vi "Sequence.BuildChannelLookup.vi"(8 "error in (no error)":errorcluster, 10 "Output Channels":T1[](array[typedef]), 11 "ChannelLookup":variant) -> (0 "error out":errorcluster, 3 "ChannelLookup":variant)   [LabVIEW 2013, in "Simple Sequence Editor.lvlib"]
uses:
  Simple Sequence Editor.lvlib
  Types/ChannelProperties.ctl
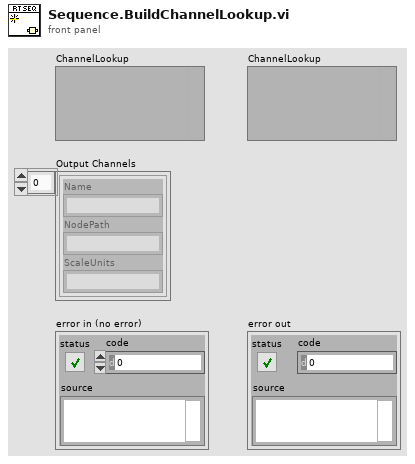
[diagram p1: front panel]
types:
  T1 = typedef "Simple Sequence Editor.lvlib/ChannelProperties.ctl" = cluster{"Name":string, "NodePath":string, "ScaleUnits":string}
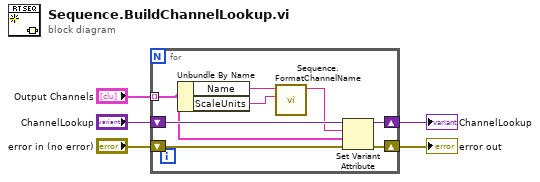
[diagram p0: block diagram]
diagram:
  n1 = for {
    shift-right: [w12] -> w5
    shift-left: "ChannelLookup" -> [w13]
    shift-right: [w11] -> w4
    shift-left: "error in (no error)" -> [w10]
    tunnel: "Output Channels" -> [w9] mode=indexing
    n2 = Unbundle By Name(w9) -> ("Name"=w7:string, "ScaleUnits"=w8:string)
    n3 = call "Sequence.FormatChannelName.vi"("ScaleUnits"=w8, "Name"=w7) -> ("String"=w6:string)  [unwired: 9 in]
    n4 = Set Variant Attribute(Variant=w13, name=w6, value=w9, error in=w10) -> (Variant out=w12:variant, error out=w11:errorcluster)  [unwired: 1 out]
  }
  "ChannelLookup" <- w5
  "error out" <- w4
